vi "test_signal2word2signal.vi"() -> ()   [LabVIEW 2020]
uses:
  Source/RT Driver/RT Driver/Controls/Asynchronous - Parameter map_type.ctl
  Source/Shared/EncodeDecode/_typedefs/parameter_config_type.ctl
  Source/Shared/EncodeDecode/_typedefs/parameter_config_type_type.ctl
  Source/Shared/EncodeDecode/_typedefs/parameter_config_encoding_type.ctl
  Source/RT Driver/Ballard MIL-1553 Engine.lvlib
panel:
  out "parameters out":dbl[](array[numeric])
  out "words out":u16[](array[numeric]) format="%016b"
  in  "parameters in":dbl[](array[numeric])
  in  "param map":T1
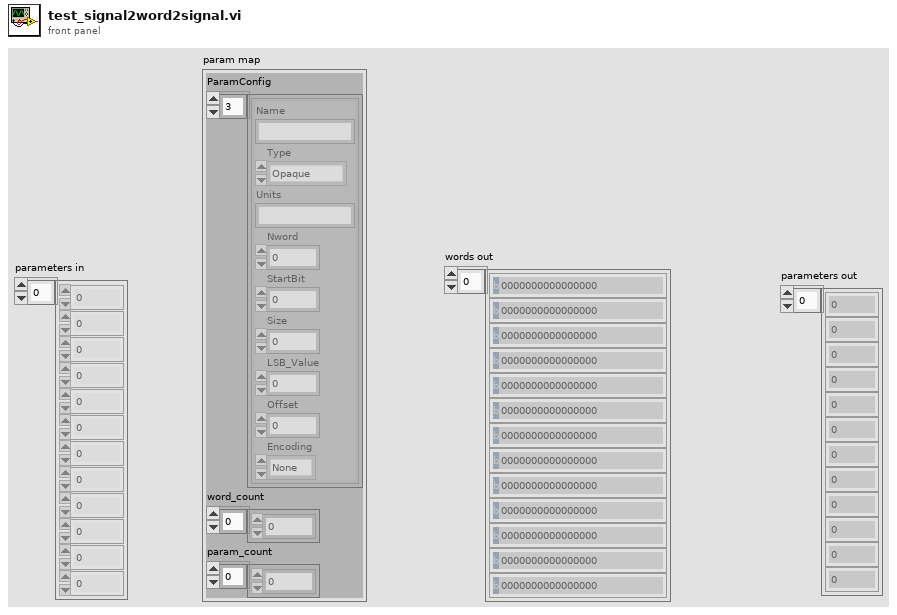
[diagram p1: front panel]
types:
  T1 = typedef "Ballard MIL-1553 Engine.lvlib/Asynchronous - Parameter map_type.ctl" = cluster{"ParamConfig":T2[], "word_count":u8[], "param_count":u8[]}
  T2 = typedef "parameter_config_type.ctl" = cluster{"Name":string, "Type":T3, "Units":string, "Nword":i32, "StartBit":i32, "Size":i32, "LSB_Value":dbl, "Offset":i32, "Encoding":T4}
  T3 = typedef "parameter_config_type_type.ctl" = enum16{"Opaque", "Enum", "Float", "Integer", "Bcd", "Bool"}
  T4 = typedef "parameter_config_encoding_type.ctl" = enum16{"None", "2-complement", "Unsigned"}
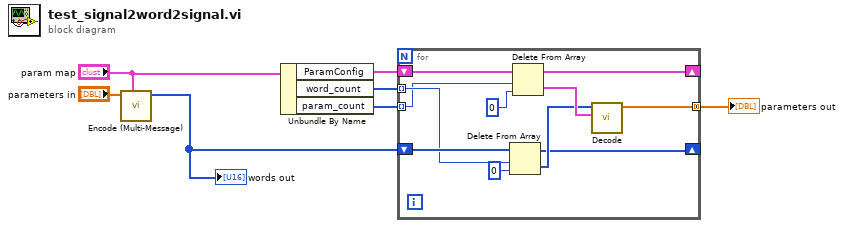
[diagram p0: block diagram]
diagram:
  n1 = call "Encode (Multi-Message).vi"("param map"="param map", "parameters in"="parameters in") -> ("words out"=w2:u16[])  [unwired: 9 in]
  "words out" <- w2
  n2 = Unbundle By Name("param map") -> ("ParamConfig"=w3:T2[], "word_count"=w5:u8[], "param_count"=w4:u8[])
  n3 = for {
    tunnel: w5 -> [w13] mode=indexing
    tunnel: w4 -> [w12] mode=indexing
    shift-right: [w17] -> _
    shift-left: w3 -> [w18]
    shift-right: [w9] -> _
    shift-left: w2 -> [w15]
    tunnel: [w8] -> w1 mode=concatenating
    n4 = Delete From Array(array=w15, length=w13, index=0) -> (deleted portion=w10:u16[], array with subset deleted=w9:u16[])
    n5 = Delete From Array(array=w18, length=w12, index=0) -> (deleted portion=w11:T2[], array with subset deleted=w17:T2[])
    n6 = call "Decode.vi"("ParamConfig"=w11, "Words In"=w10) -> ("Parameters out"=w8:dbl[])  [unwired: 9 in]
  }
  "parameters out" <- w1
